vi "Sync Diagonal Cursor Mask Plot.vi"(10 "Cursor Mask":refnum<vi>, 11 "Freq-RPM Map":refnum<vi>) -> (1 "diagonal line":cluster{dbl, dbl}[](array[cluster]) {"?" format="%.2f"; "?" format="%.2f"}, 2 "order number":dbl format="%.2f", 3 "Cursor Position":cluster{"Cursor X":dbl, "Cursor Y":dbl} {"Cursor Y" format="%.2f"; "Cursor X" format="%.2f"})   [LabVIEW 2017]
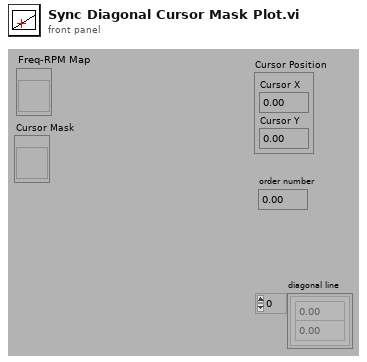
[diagram p1: front panel]
types:
  T1 = typedef "LVRangeTypeDef.ctl" = cluster{"Minimum":dbl, "Maximum":dbl, "Increment":dbl, "Minor Increment":dbl, "Start":dbl}
  T2 = typedef "LVPointDoubleTypeDef.ctl" = cluster{"Cursor X":dbl, "Cursor Y":dbl}
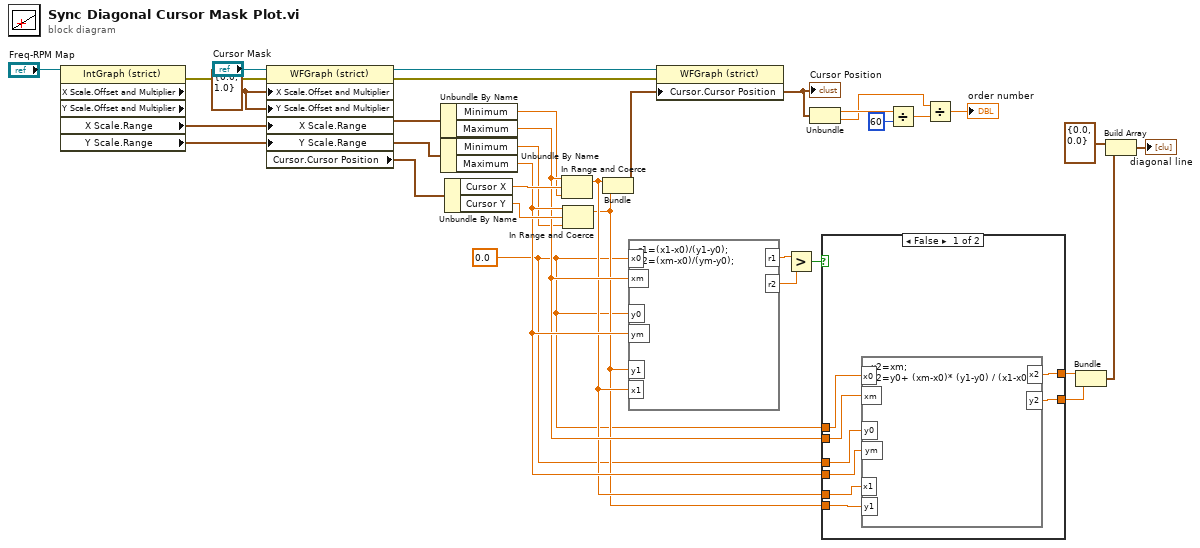
[diagram p0: block diagram]
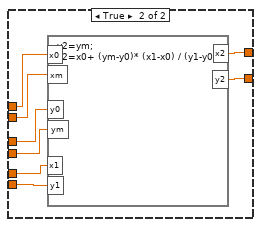
[diagram p2: hidden frame]
diagram:
  w7 = 0.0 ("Input Variable")
  w11 = cluster{"Offset":dbl, "Multiplier":dbl} {"Offset"=0.0, "Multiplier"=1.0} ("X Scale.Offset and Multiplier")
  n1 = property on="Property Node" class="IntGraph (strict)" props=["X Scale", "Offset and Multiplier", "Y Scale", "Offset and Multiplier", "X Scale", "Range", "Y Scale", "Range"](reference="Freq-RPM Map") -> (error out=w24:errorcluster, "X Scale.Range"=w30:T1, "Y Scale.Range"=w29:T1)  [unwired: 1 in, 3 out]
  n2 = property on="Property Node" class="WFGraph (strict)"(reference="Cursor Mask", error in=w24, "X Scale.Offset and Multiplier"=w11, "Y Scale.Offset and Multiplier"=w11, "X Scale.Range"=w30, "Y Scale.Range"=w29) -> (reference out=w25:refnum<vi>, error out=w23:errorcluster, "Cursor.Cursor Position"=w28:T2)
  n3 = Unbundle By Name(w30) -> ("Minimum"=w9:dbl, "Maximum"=w18:dbl)
  n4 = Unbundle By Name(w29) -> ("Minimum"=w8:dbl, "Maximum"=w19:dbl)
  n5 = Unbundle By Name(w28) -> ("Cursor X"=w27:dbl, "Cursor Y"=w26:dbl)
  n6 = In Range and Coerce(upper limit=w18, x=w27, lower limit=w9) -> (coerced(x)=w17:dbl)  [unwired: 1 out]
  n7 = In Range and Coerce(upper limit=w19, x=w26, lower limit=w8) -> (coerced(x)=w16:dbl)  [unwired: 1 out]
  n8 = Bundle("Maximum"=w17, "Maximum"=w16) -> (w6:cluster{"Maximum":dbl, "Maximum":dbl})  [unwired: 1 in]
  "Cursor Position" <- w6
  n9 = formula code="r1=(x1-x0)/(y1-y0);\nr2=(xm-x0)/(ym-y0);"("x0"=w7, "y0"=w7, "x1"=w17, "y1"=w16, "xm"=w18, "ym"=w19) -> ("r1"=w22:dbl, "r2"=w21:dbl)
  n10 = property on="Property Node" class="WFGraph (strict)"(reference=w25, error in=w23, "Cursor.Cursor Position"=w6) -> ()  [unwired: 2 out]
  n11 = Greater?(x=w22, y=w21) -> (0:w20:bool)
  n12 = Unbundle(w6) -> ("Maximum"=w5:dbl, "Maximum"=w2:dbl)
  n13 = case shown="False" w20 {
    tunnel: w19 -> [w35 w45]
    tunnel: w7 -> [w36 w46]
    tunnel: w7 -> [w38 w48]
    tunnel: w18 -> [w37 w47]
    tunnel: w17 -> [w34 w44]
    tunnel: w16 -> [w33 w43]
    tunnel: [w40 w42] -> w15
    tunnel: [w39 w41] -> w14
    frame False {
      n14 = formula code="x2=xm;\ny2=y0+ (xm-x0)* (y1-y0) / (x1-x0);"("x0"=w38, "y0"=w36, "y1"=w33, "x1"=w34, "xm"=w37, "ym"=w35) -> ("x2"=w40:dbl, "y2"=w39:dbl)
    }
    frame True {
      n15 = formula code="y2=ym;\nx2=x0+ (ym-y0)* (x1-x0) / (y1-y0);"("x0"=w48, "y0"=w46, "y1"=w43, "x1"=w44, "xm"=w47, "ym"=w45) -> ("x2"=w42:dbl, "y2"=w41:dbl)
    }
  }
  n16 = Divide(x=w5, y=60) -> (x/y=w3:dbl)
  n17 = Divide(x=w2, y=w3) -> (x/y=→"order number":dbl)
  n18 = Bundle("x2"=w15, "y2"=w14) -> (w13:cluster{"x2":dbl, "y2":dbl})  [unwired: 1 in]
  n19 = Build Array(cluster{"x2":dbl, "y2":dbl} {"x2"=0.0, "y2"=0.0} ("Input Element"), w13) -> (→"diagonal line":cluster{"x2":dbl, "y2":dbl}[])
